vi "Segment n Coder.vi"(9 "Segment 1 to 99":T1(array[cluster]), 10 "File ID":string, 11 "仪器地址":u32) -> (3 "Output":string[](array[string]))   [LabVIEW 2010, in "DCP551.lvlib"]
uses:
  DCP551.lvlib
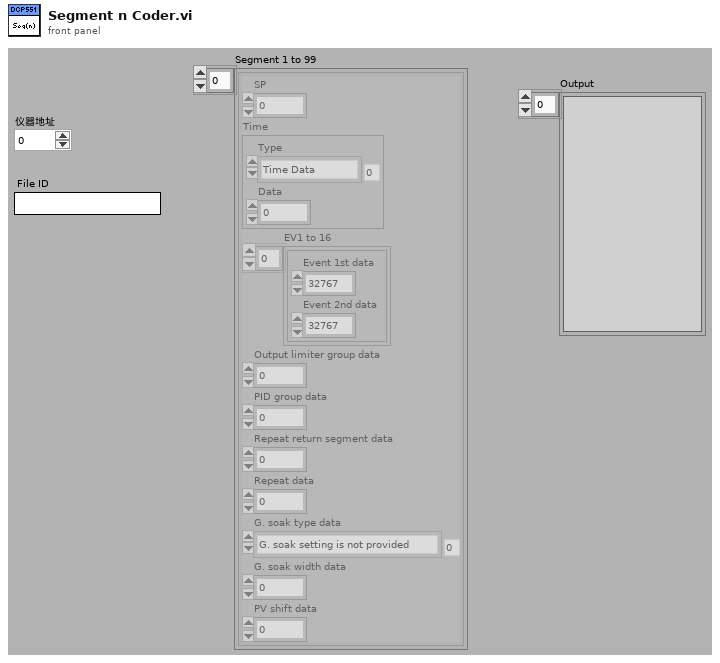
[diagram p1: front panel]
types:
  T1 = cluster{"SP":dbl, "Time":cluster{"Type":enum16{"Time Data", "delta Dtada", "SP Data"}, "Data":i32}, "EV1 to 16":cluster{"Event 1st data":i32, "Event 2nd data":i32}[], "Output limiter group data":i32, "PID group data":i32, "Repeat return segment data":i32, "Repeat data":i32, "G. soak type data":enum16{"G. soak setting is not provided", "Segment start point", "Segment end point", "Total segment"}, "G. soak width data":i32, "PV shift data":i32}[]
  T2 = cluster{"Event 1st data":i32, "Event 2nd data":i32}[]
  T3 = enum16{"G. soak setting is not provided", "Segment start point", "Segment end point", "Total segment"}
  T4 = cluster{"Event 1st data":i32, "Event 2nd data":i32}
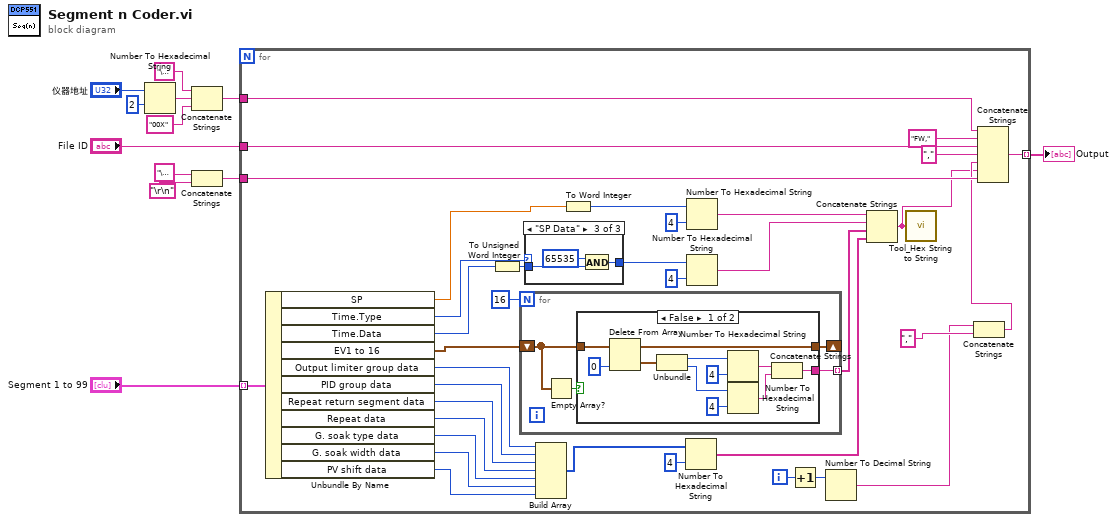
[diagram p0: block diagram]
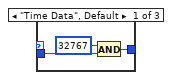
[diagram p2: hidden frame]
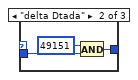
[diagram p3: hidden frame]
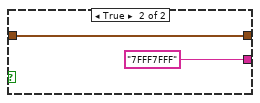
[diagram p4: hidden frame]
diagram:
  n1 = Number To Hexadecimal String(1:i16 2 ("width (-)"), 2:"仪器地址") -> (0:w9:string)
  n2 = Concatenate Strings("\u0002" ("string"), w9, "00X" ("string")) -> (w4:string)
  n3 = Concatenate Strings("\u0003" ("string"), "\r\n") -> (w2:string)
  n4 = for {
    tunnel: "Segment 1 to 99" -> [w48] mode=indexing
    tunnel: [w18] -> w1 mode=indexing
    tunnel: w4 -> [w25]
    tunnel: "File ID" -> [w23]
    tunnel: w2 -> [w19]
    i -> [w20]
    n5 = Unbundle By Name(w48) -> ("SP"=w13:dbl, "Time.Type"=w46:enum16{"Time Data", "delta Dtada", "SP Data"}, "Time.Data"=w45:i32, "EV1 to 16"=w47:T2, "Output limiter group data"=w34:i32, "PID group data"=w33:i32, "Repeat return segment data"=w32:i32, "Repeat data"=w31:i32, "G. soak type data"=w30:T3, "G. soak width data"=w29:i32, "PV shift data"=w28:i32)
    n6 = To Unsigned Word Integer(number=w45) -> (unsigned 16bit integer=w44:u16)
    n7 = for {
      N: 16 -> [_]
      shift-right: [w61] -> _
      shift-left: w47 -> [w60]
      tunnel: [w58] -> w26 mode=indexing
      n8 = Empty Array?(array=w60) -> (empty?=w59:bool)
      n9 = case shown="False" w59 {
        tunnel: [w66 w74] -> w61
        tunnel: w60 -> [w65 w74]
        tunnel: [w62 "7FFF7FFF"] -> w58
        frame False {
          n10 = Delete From Array(array=w65, index=0) -> (deleted portion=w67:T4, array with subset deleted=w66:T2)  [unwired: 1 in]
          n11 = Unbundle(w67) -> ("Event 1st data"=w71:i32, "Event 2nd data"=w69:i32)
          n12 = Number To Hexadecimal String(1:i16 4 ("width (-)"), 2:w71) -> (0:w64:string)
          n13 = Number To Hexadecimal String(1:i16 4 ("width (-)"), 2:w69) -> (0:w63:string)
          n14 = Concatenate Strings(w64, w63) -> (w62:string)
        }
        frame True {
        }
      }
    }
    n15 = case shown="\"SP Data\"" w46 {
      tunnel: w44 -> [w50 w53 w56]
      tunnel: [w49 w52 w55] -> w41
      frame "Time Data", Default {
        n16 = And(x=u16 32767, y=w50) -> (x .and. y?=w49:u16)
      }
      frame "delta Dtada" {
        n17 = And(x=u16 49151, y=w53) -> (x .and. y?=w52:u16)
      }
      frame "SP Data" {
        n18 = And(x=u16 65535, y=w56) -> (x .and. y?=w55:u16)
      }
    }
    n19 = Build Array(w34, w33, w32, w31, w30, w29, w28) -> (w27:i32[])
    n20 = To Word Integer(number=w13) -> (16bit integer=w43:i16)
    n21 = Number To Hexadecimal String(1:i16 4 ("width (-)"), 2:w27) -> (0:w35:string[])
    n22 = Number To Hexadecimal String(1:i16 4 ("width (-)"), 2:w43) -> (0:w40:string)
    n23 = Number To Hexadecimal String(1:i16 4 ("width (-)"), 2:w41) -> (0:w39:string)
    n24 = Increment(x=w20) -> (x+1=w21:i32)
    n25 = Number To Decimal String(number=w21) -> (decimal integer string=w16:string)  [unwired: 1 in]
    n26 = Concatenate Strings(w40, w39, w26, w35) -> (w14:string)
    n27 = call "Tool_Hex String to String.vi"("Hex String"=w14) -> ()  [unwired: 14 in, 1 out]
    n28 = Concatenate Strings(w16, "," ("string")) -> (w15:string)
    n29 = Concatenate Strings(w25, "FW," ("string"), w23, "," ("string"), w15, w14, w19) -> (w18:string)
  }
  "Output" <- w1
